vi "Gergberg Image Manipulation.vi"() -> ()   [LabVIEW 2012, in "LightPipes.lvlib"]
uses:
  LightPipes.lvlib
  <vilib>/vision/NI_Vision_Development_Module.lvlib
panel:
  in  "Image Type":T1=7 items=["Grayscale (U8)", "Grayscale (I16)", "Grayscale (SGL)", "Complex (CSG)", "RGB (U32)", "HSL (U32)", "RGB (U64)", "Grayscale (U16)"]
  in  "FF Resolution  (micron/pix)":dbl=2.96
  in  "Final Resolution  (micron/pix)":dbl=2.96
  out "MF Original":cluster{"X Resolution":i32, "Y Resolution":i32}={"X Resolution"=1115, "Y Resolution"=1191}
  out "FF Original":cluster{"X Resolution":i32, "Y Resolution":i32}={"X Resolution"=640, "Y Resolution"=480}
  in  "stop":bool
  out "MF":T2(plugin-control)
  out "FF":T2(plugin-control)
  in  "Balance Energy":bool=TRUE
  in  "MF Rotate 180":bool=TRUE
  in  "MF Resolution (micron/pix)":dbl=7.38
  in  "Final Size (pix)":i32=300 step=10
  in  "Run":bool
  in  "Save MF":bool
  out "FF Current":cluster{"X Resolution":i32, "Y Resolution":i32}={"X Resolution"=300, "Y Resolution"=300}
  out "MF Current":cluster{"X Resolution":i32, "Y Resolution":i32}={"X Resolution"=300, "Y Resolution"=300}
  in  "Save FF":bool
  in  "Mid Field":path=path "C:/Users/Tri/Documents/Lightpipes/LabView/beam images/MF Masked.png"
  in  "Far Field":path=path "C:/Users/Tri/Documents/Lightpipes/LabView/beam images/FF Masked.png"
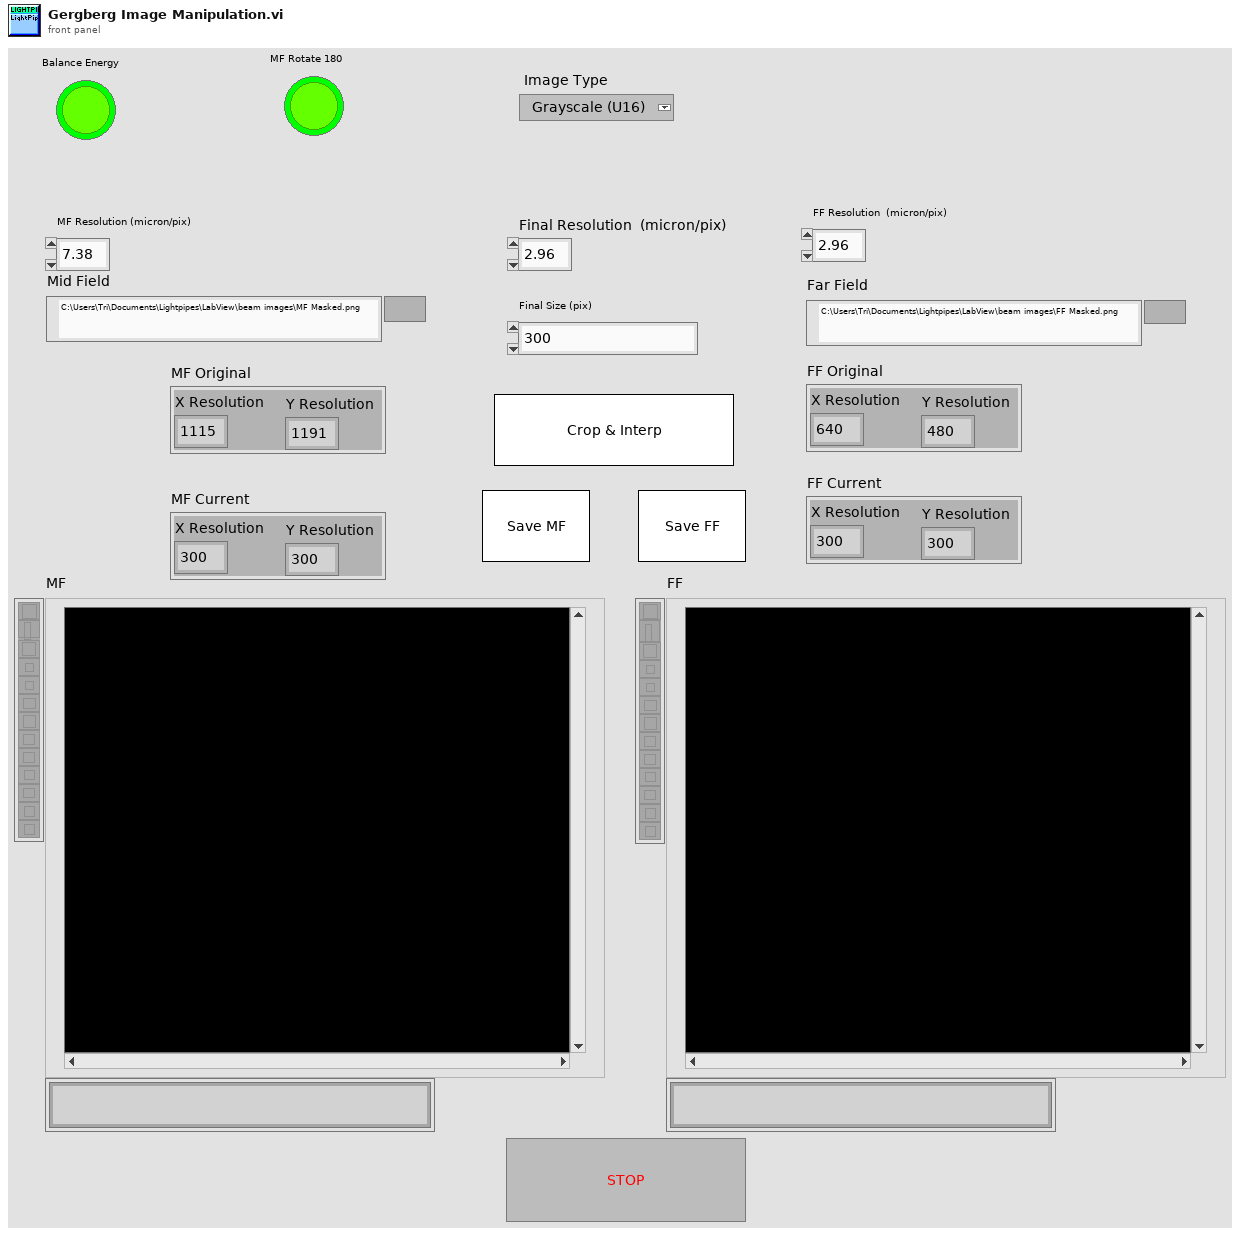
[diagram p1: front panel]
types:
  T1 = typedef "Image Type" = u32
  T2 = typedef "IMAQ Image.ctl" = refnum<image>
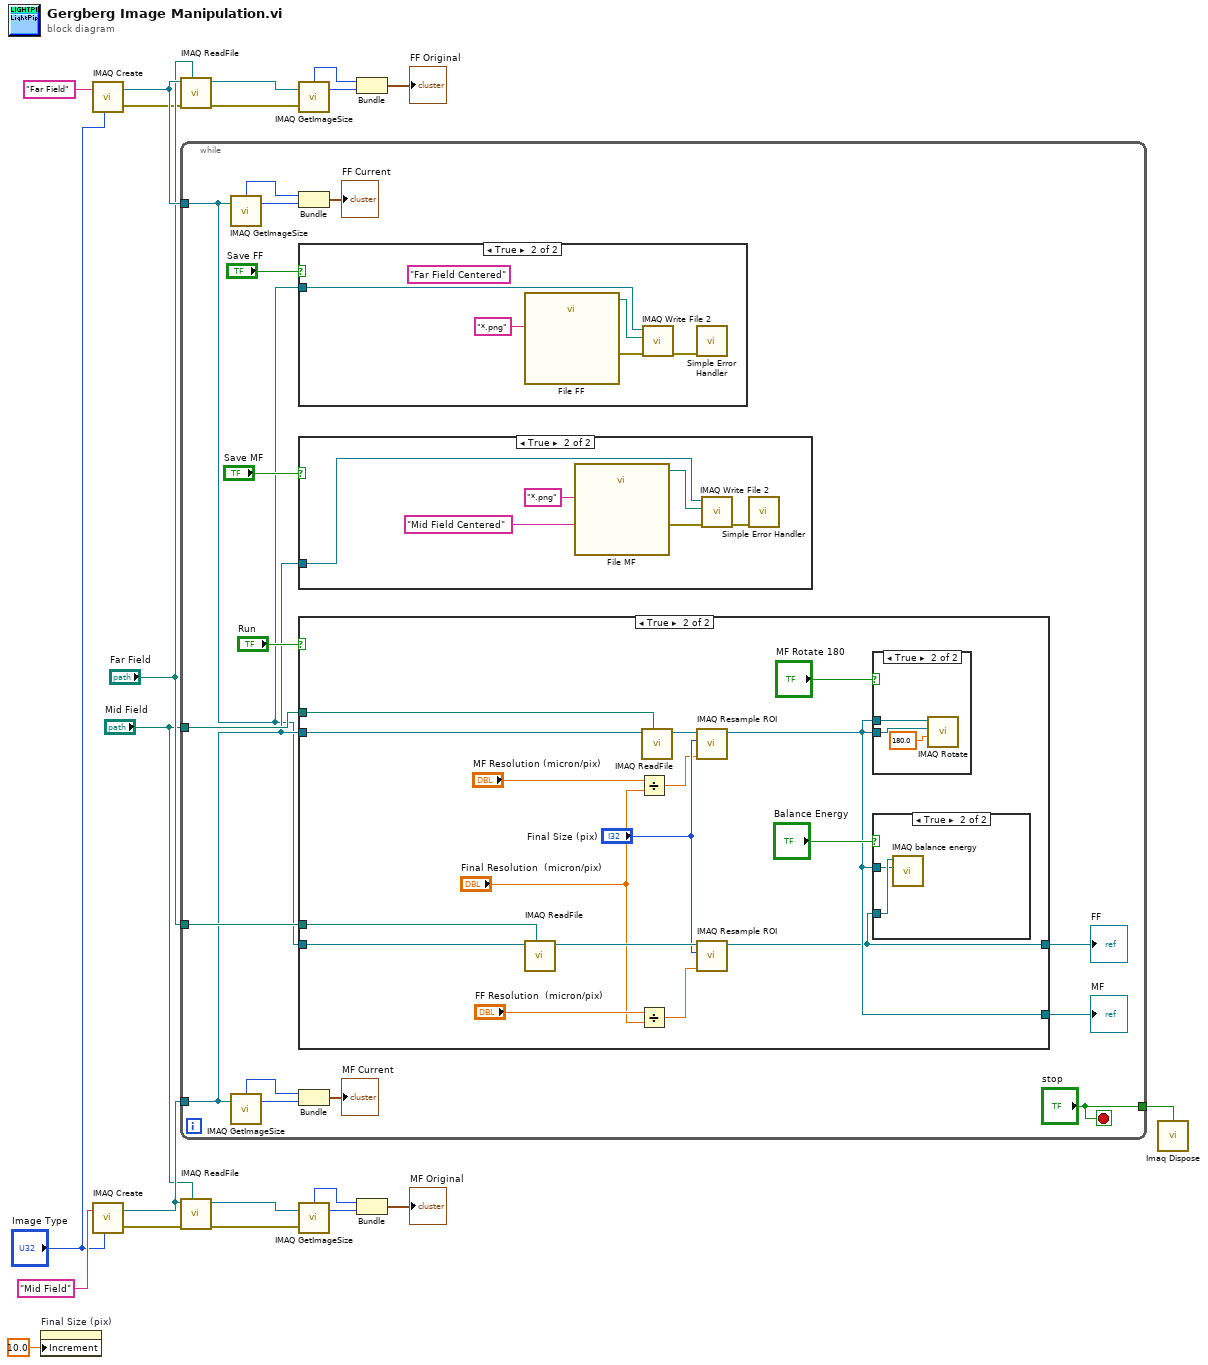
[diagram p0: block diagram]
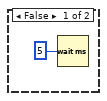
[diagram p3: hidden frame]
diagram:
  n1 = property on="Final Size (pix)" class="DigNum (strict)"("Increment"=10.0 ("Data Entry Limits:Increment")) -> ()  [unwired: 2 in, 2 out]
  n2 = call "IMAQ Create"("Image Name"="Far Field", "Image Type"="Image Type") -> ("New Image"=w18:T2, "error out"=w6:errorcluster)  [unwired: 3 in]
  n3 = call "IMAQ Create"("Image Name"="Mid Field", "Image Type"="Image Type") -> ("New Image"=w16:T2, "error out"=w5:errorcluster)  [unwired: 3 in]
  n4 = call "IMAQ ReadFile"("File Path"="Far Field", "error in (no error)"=w6, "Image"=w18) -> ("error out"=w7:errorcluster, "Image Out"=w4:T2)  [unwired: 2 in, 5 out]
  n5 = while {
    tunnel: "Far Field" -> [w37]
    tunnel: w18 -> [w25]
    tunnel: "Mid Field" -> [w36]
    tunnel: w16 -> [w27]
    tunnel: ["stop"] -> w2
    stop <- "stop" stop-if-true
    n6 = call "IMAQ GetImageSize"("Image"=w25) -> ("Y Resolution"=w32:i32, "X Resolution"=w31:i32)  [unwired: 3 in, 1 out]
    n7 = call "IMAQ GetImageSize"("Image"=w27) -> ("Y Resolution"=w29:i32, "X Resolution"=w28:i32)  [unwired: 3 in, 1 out]
    n8 = Bundle("X Resolution"=w31, "Y Resolution"=w32) -> (→"FF Current":cluster{"X Resolution":i32, "Y Resolution":i32})  [unwired: 1 in]
    n9 = case shown="True" "Save FF" {
      tunnel: w25 -> [_ w40]
      frame False {
      }
      frame True {
        (unwired) "Far Field Centered" ("default name")
        n10 = call "File FF"("pattern (all files)"="*.png") -> ("selected path"=w42:path, "error out"=w41:errorcluster)  [unwired: 11 in, 2 out]
        n11 = call-poly "IMAQ Write File 2"("error in (no error)"=w41, "File Path"=w42, "Image"=w40) -> ("error out"=w39:errorcluster)  [unwired: 7 in, 1 out]
        n12 = call <vilib>:"Simple Error Handler.vi"("error in (no error)"=w39) -> ()  [unwired: 4 in, 5 out]
      }
    }
    n13 = case shown="True" "Save MF" {
      tunnel: w27 -> [_ w48]
      frame False {
        n14 = Wait (ms)(milliseconds to wait=u32 5) -> ()  [unwired: 1 out]
      }
      frame True {
        n15 = call "File MF"("prompt"="Mid Field Centered" ("default name"), "pattern (all files)"="*.png") -> ("selected path"=w49:path, "error out"=w45:errorcluster)  [unwired: 10 in, 2 out]
        n16 = call-poly "IMAQ Write File 2"("error in (no error)"=w45, "File Path"=w49, "Image"=w48) -> ("error out"=w44:errorcluster)  [unwired: 7 in, 1 out]
        n17 = call <vilib>:"Simple Error Handler.vi"("error in (no error)"=w44) -> ()  [unwired: 4 in, 5 out]
      }
    }
    n18 = case shown="True" "Run" {
      tunnel: w37 -> [_ w67]
      tunnel: w25 -> [w50 w66]
      tunnel: w36 -> [_ w65]
      tunnel: w27 -> [w51 w62]
      tunnel: [w51 w53] -> w24
      tunnel: [w50 w52] -> w23
      frame False {
      }
      frame True {
        n19 = call "IMAQ ReadFile"("File Path"=w67, "Image"=w66) -> ("Image Out"=w60:T2)  [unwired: 3 in, 6 out]
        n20 = Divide(x="MF Resolution (micron/pix)", y="Final Resolution  (micron/pix)") -> (x/y=w57:dbl)
        n21 = Divide(x="FF Resolution  (micron/pix)", y="Final Resolution  (micron/pix)") -> (x/y=w58:dbl)
        n22 = call "IMAQ ReadFile"("File Path"=w65, "Image"=w62) -> ("Image Out"=w61:T2)  [unwired: 3 in, 6 out]
        n23 = call "IMAQ Resample ROI.vi"("Interp Ratio"=w57, "Final Size"="Final Size (pix)", "Image In"=w61) -> ("Image Out"=w53:T2)  [unwired: 8 in]
        n24 = call "IMAQ Resample ROI.vi"("Interp Ratio"=w58, "Final Size"="Final Size (pix)", "Image In"=w60) -> ("Image Out"=w52:T2)  [unwired: 8 in]
        n25 = case shown="True" "MF Rotate 180" {
          tunnel: w53 -> [_ w69]
          tunnel: w53 -> [_ w68]
          frame False {
          }
          frame True {
            n26 = call "IMAQ Rotate"("Angle (degrees)"=sgl 180.0, "Image Dst"=w68, "Image Src"=w69) -> ()  [unwired: 7 in, 2 out]
          }
        }
        n27 = case shown="True" "Balance Energy" {
          tunnel: w53 -> [_ w71]
          tunnel: w52 -> [_ w72]
          frame False {
          }
          frame True {
            n28 = call "IMAQ balance energy.vi"("Target Image"=w71, "Base Image"=w72) -> ()  [unwired: 9 in, 1 out]
          }
        }
      }
    }
    "MF" <- w24
    "FF" <- w23
    n29 = Bundle("X Resolution"=w28, "Y Resolution"=w29) -> (→"MF Current":cluster{"X Resolution":i32, "Y Resolution":i32})  [unwired: 1 in]
  }
  n30 = call "IMAQ ReadFile"("File Path"="Mid Field", "error in (no error)"=w5, "Image"=w16) -> ("error out"=w8:errorcluster, "Image Out"=w1:T2)  [unwired: 2 in, 5 out]
  n31 = call "IMAQ GetImageSize"("Image"=w4, "error in (no error)"=w7) -> ("Y Resolution"=w13:i32, "X Resolution"=w14:i32)  [unwired: 2 in, 1 out]
  n32 = call "IMAQ GetImageSize"("Image"=w1, "error in (no error)"=w8) -> ("Y Resolution"=w9:i32, "X Resolution"=w10:i32)  [unwired: 2 in, 1 out]
  n33 = Bundle("X Resolution"=w14, "Y Resolution"=w13) -> (→"FF Original":cluster{"X Resolution":i32, "Y Resolution":i32})  [unwired: 1 in]
  n34 = Bundle("X Resolution"=w10, "Y Resolution"=w9) -> (→"MF Original":cluster{"X Resolution":i32, "Y Resolution":i32})  [unwired: 1 in]
  n35 = call "Imaq Dispose"("All Images? (No)"=w2) -> ()  [unwired: 5 in, 1 out]
